vi "WPI_IMU_ADIS16448_ReadRegister.vi"(8 "error in (no error)":errorcluster, 10 "Register":u8, 11 "SPIDevRef in":T1) -> (0 "error out":errorcluster, 2 "Register Value":u16, 3 "SPIDevRef out":T1)   [LabVIEW 2015, in "FRC ADI MXP IMU.lvlib"]
uses:
  FRC ADI MXP IMU.lvlib
  <vilib>/Rock Robotics/WPI/SPI/WPI_SPIDevRef.ctl
  <vilib>/Rock Robotics/SystemInterfaces/spilib/spi_bus.ctl
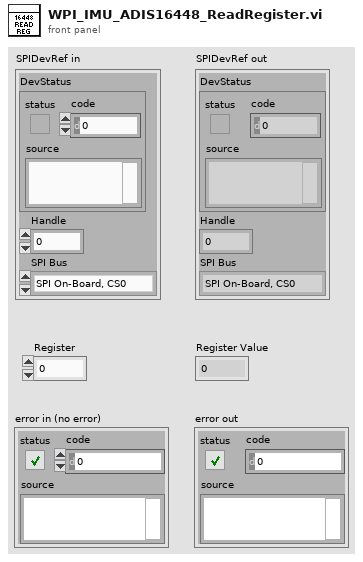
[diagram p1: front panel]
types:
  T1 = typedef "WPI_SPIDevRef.ctl" = cluster{"DevStatus":errorcluster, "Handle":i32, "SPI Bus":T2}
  T2 = typedef "spi_bus.ctl" = enum16{"SPI On-Board, CS0", "SPI On-Board, CS1", "SPI On-Board, CS2", "SPI On-Board, CS3", "SPI MXP", "Invalid"}
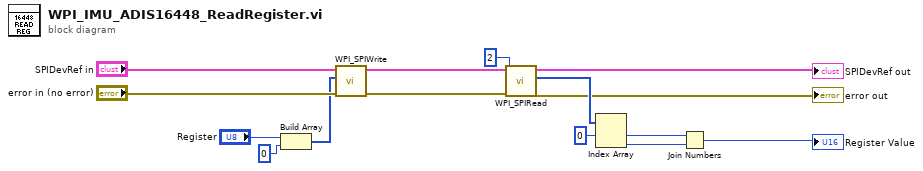
[diagram p0: block diagram]
diagram:
  n1 = Build Array("Register", u8 0 ("element")) -> (w5:u8[])
  n2 = call <vilib>:"WPI_SPIWrite.vi"("error in (no error)"="error in (no error)", "Data To Send"=w5, "SPIDevRef"="SPIDevRef in") -> ("error out"=w1:errorcluster, "SPIDevRef"=w11:T1)  [unwired: 7 out]
  n3 = call <vilib>:"WPI_SPIRead.vi"("error in (no error)"=w1, "Num to Read"=2, "SPIDevRef"=w11) -> ("error out"=→"error out":errorcluster, "Received Data"=w9:u8[], "SPIDevRef"=→"SPIDevRef out":T1)  [unwired: 6 in]
  n4 = Index Array(array=w9, index #1=0 ("index")) -> (element #1=w3:u8, element #2=w2:u8)  [unwired: 1 in]
  n5 = Join Numbers(hi=w3, lo=w2) -> ((hi.lo)=→"Register Value":u16)
